vi "Create Reply Queue.vi"(8 "error in (no error)":errorcluster) -> (0 "error out":errorcluster, 3 "Reply Queue Out":refnum<queue>)   [LabVIEW 2015, in "Broadcast Actor.lvlib" / "Broadcast Actor.lvclass"]
uses:
  Broadcast Actor.lvclass
  Type Defs/Events Type Def.ctl
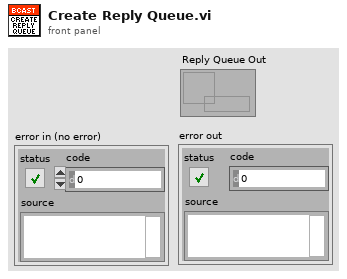
[diagram p1: front panel]
types:
  T1 = typedef "Broadcast Actor.lvlib/Broadcast Actor.lvclass/Events Type Def.ctl" = cluster{"Error Event":refnum<user-event>}
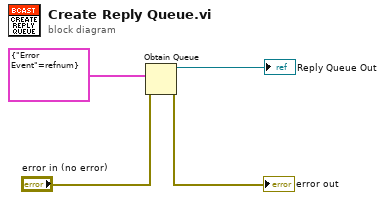
[diagram p0: block diagram]
diagram:
  n1 = Obtain Queue(element data type=T1 {"Error Event"=refnum} ("Events"), error in (no error)="error in (no error)") -> (queue out=→"Reply Queue Out":refnum<queue>, error out=→"error out":errorcluster)  [unwired: 3 in, 1 out]
